vi "DisplacementLogic.vi"   [LabVIEW 2016]
uses:
  DisplacementData.ctl
  DisplacementStates.ctl
  <vilib>/Platform/TimedLoop/XDataNode/timing_clust.ctl
  <vilib>/Platform/TimedLoop/XDataNode/nitl_modes.ctl
  <vilib>/Platform/TimedLoop/XDataNode/wakeup.ctl
  Telemetry/TelemetryFields.ctl
  Telemetry/TelemetryDataTypes.ctl
  Telemetry/TelemetryUpdateModes.ctl
  DisplacementErrorCodes.ctl
  <vilib>/rvi/Emulation/niFpgaSctlEmulationGetInTimedLoop.vi
  <vilib>/rvi/Emulation/niFpgaEmulationReportErrorSimple.vi
  <vilib>/rvi/Emulation/niFpgaGetClockAttributes.vi
  <vilib>/rvi/Emulation/niFpgaCriticalErrorInLSC.vi
  <vilib>/rvi/Emulation/niFpgaEmulationIsFPGAContextNoSignature.vi
  <vilib>/rvi/DataTransferAndStorage/Container/Common/niFpgaContainerGetUniqueNameForEmu.vi
  <vilib>/rvi/Memory/Memory_Emulation/niFpgaMemoryEmulationCacheClearOnFirstRun.vi
  <vilib>/rvi/Memory/Memory_Emulation/nirvimemoryEmulationManagerCache_MakeExclusive.vi
  <vilib>/rvi/Memory/Memory_Emulation/niFpgaMemoryEmulationValidateCache.vi
  <vilib>/rvi/Memory/Memory_Emulation/nirvimemoryEmulationManagerCache_InsertValue.vi
  <vilib>/Utility/error.llb/Clear Errors.vi
  <vilib>/rvi/Memory/Memory_Emulation/nirvimemoryEmulationManagerCache_ReleaseExclusive.vi
  <vilib>/rvi/Memory/Memory_Emulation/nirvimemoryEmulationManagerCache_GetValue.vi
  <vilib>/rvi/Memory/Memory_Emulation/nirvimemoryEmulationManagerCache_SetValue.vi
  <vilib>/rvi/Emulation/niFpgaProcessEmulError.vi
  <vilib>/rvi/errors/niFpgaSetErrorForExecOnDevCompSimple.vi
  <vilib>/rvi/eio/common/nirviEmuReportErrorAndStop.vi
  <vilib>/rvi/FIFO/Fifo_Resource/nirvififoEmulationSetSize.vi
  <vilib>/rvi/FIFO/Fifo_Resource/nirviFifoEmulationQueueMgr.vi
  <instcachedir>/0/nirviFifoEmulationQueueMgr_E5CAEC123FF24DC58D834DCA3CDAA9B5.lvgen/nirviFifoEmulationQueueMgr_E5CAEC123FF24DC58D834DCA3CDAA9B5_009.vi
  <vilib>/rvi/FIFO/Fifo_Resource/nirvififoEmulationDetermineInputValidOut.vi
  <vilib>/rvi/FIFO/Fifo_Resource/nirvififoEmulationCreateLock.vi
  <vilib>/rvi/FIFO/Fifo_Resource/nirvififoEmulationObtainLock.vi
  <vilib>/rvi/FIFO/Fifo_Resource/nirvififoEmulationReleaseLock.vi
  <vilib>/rvi/occurrence/nirviWaitOnOccurrenceBase.vi
  <vilib>/rvi/errors/nirviReportUnexpectedCaseInternalError.vi
  <vilib>/rvi/errors/nirviReportUnexpectedCaseInternalError (U32).vi
  <instcachedir>/0/nirviFifoEmulationQueueMgr_E5CAEC123FF24DC58D834DCA3CDAA9B5.lvgen/nirviFifoEmulationQueueMgr_E5CAEC123FF24DC58D834DCA3CDAA9B5_024.vi
  <vilib>/rvi/eio/common/nirviEmuTemplateMethod_errors.vi
  <vilib>/Platform/TimedLoop/XDataNode/XDataNode.xnode
  <vilib>/rvi/DataTransferAndStorage/Container/XNode/niFpgaContainer.xnode
  <vilib>/rvi/DataTransferAndStorage/Register/Emulation/niFpgaRegisterEmulation.vi
  <vilib>/rvi/FIFO/Fifo_Resource/nirvififoEmulationWrite.vi
  <vilib>/rvi/FIFO/Fifo_Resource/nirvififoEmulationRead.vi
  <vilib>/eio/EIONode/EIONode.xnode
  <vilib>/Platform/TimedLoop/XDataNode/XDNodeRunTimeDep.lvlib
types:
  T1 = typedef "DisplacementData.ctl" = cluster{"State":T2, "Flags":u8, "Sensor":u8, "Timestamp":u64, "Negative":bool, "Sensor1":i32, "Sensor2":i32, "Sensor3":i32, "Sensor4":i32, "Sensor5":i32, "Sensor6":i32, "Sensor7":i32, "Sensor8":i32}
  T2 = typedef "DisplacementStates.ctl" = enum16{"WaitForTrigger", "ClearRxFIFO", "WaitForClearComplete", "WriteM", "Write0", "WriteCR", "WriteNL", "ReadFirstCharacter", "ReadDataResponse", "ReadDeliminator", "ReadSign", "ReadHundreds", "ReadTens", "ReadOnes", "ReadDecimal", "ReadTenths", "ReadHundredths", "ReadThousandths", "ReadTenThousandths", "StartMoveData", "MoveTimestamp", "MoveData", "ReadErrorResponse", "ResponseUnknownError", "ResponseInvalidError"}
  T3 = typedef "XDNodeRunTimeDep.lvlib/timing_clust.ctl" = cluster{"Expected End [f-1]":u64, "Actual End [f-1]":u64, "Finished Late? [f-1]":bool, "Expected End [i-1]":u64, "Actual End [i-1]":u64, "Finished Late? [i-1]":bool, "Expected Start [i]":u64, "Actual Start [i]":u64, "Expected Start [f]":u64, "Actual Start [f]":u64, "Source Name":string, "Structure Name":string, "Period":i64, "Deadline":i64, "Offset":i64, "Start":i64, "Priority":i32, "Timeout":i32, "Mode":T4, "Wakeup Reason":T5, "Error":errorcluster, "Source Type":string, "Secondary Source Type":string, "Global End Time":u64, "Global Start Time":u64, "Frame Duration":u64, "Iteration Duration":u64, "Assigned CPU":i32, "I/O Scan Engine Mode":u32}
  T4 = typedef "XDNodeRunTimeDep.lvlib/nitl_modes.ctl" = enum32{"No Change", "Process missed periods, maintain original phase", "Discard missed periods, maintain original phase", "Process missed periods, ignore original phase", "Discard missed periods, ignore original phase"}
  T5 = typedef "XDNodeRunTimeDep.lvlib/wakeup.ctl" = enum32{"Normal", "Aborted", "Asynchronous wakeup", "Timing source error", "Timed loop error", "Timeout"}
  T6 = typedef "TelemetryUpdateModes.ctl" = enum8{"=", "+", "-", "|"}
  T7 = typedef "TelemetryDataTypes.ctl" = enum8{"U8", "U16", "U32", "U64", "I8", "I16", "I32", "I64", "SGL"}
  T8 = typedef "TelemetryFields.ctl" = enum16{"InclinometerErrorCode", "InclinometerTxBytes", "InclinometerRxBytes", "InclinometerTxFrames", "InclinometerRxFrames", "InclinometerTimestamp", "InclinometerAngle", "DisplacementErrorCode", "DisplacementTxBytes", "DisplacementRxBytes", "DisplacementTxFrames", "DisplacementRxFrames", "DisplacementTimestamp", "Displacement1", "Displacement2", "Displacement3", "Displacement4", "Displacement5", "Displacement6", "Displacement7", "Displacement8", "AccelerometerSampleCount", "AccelerometerTimestamp", "AccelerometerRaw1", "AccelerometerRaw2", "AccelerometerRaw3", "AccelerometerRaw4", "AccelerometerRaw5", "AccelerometerRaw6", "AccelerometerRaw7", "AccelerometerRaw8", "AccelerometerEng1", "AccelerometerEng2", "AccelerometerEng3", "AccelerometerEng4", "AccelerometerEng5", "AccelerometerEng6", "AccelerometerEng7", "AccelerometerEng8", "AngularAccelerationX", "AngularAccelerationY", "AngularAccelerationZ"}
  T9 = typedef "TelemetryUpdateData.ctl" = cluster{"DataType":T7, "Mode":T6, "Field":T8, "Data":u64}
  T10 = typedef "DisplacementErrorCodes.ctl" = u8
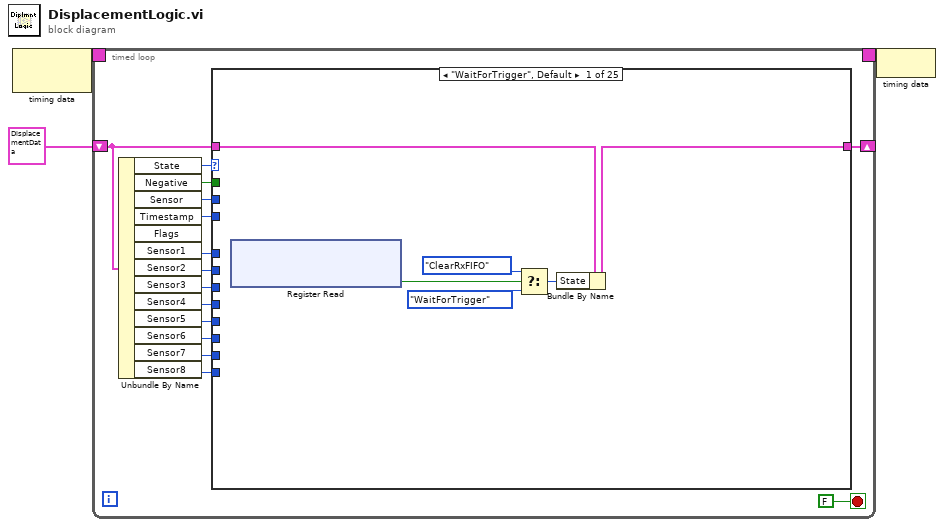
[diagram p0: block diagram]
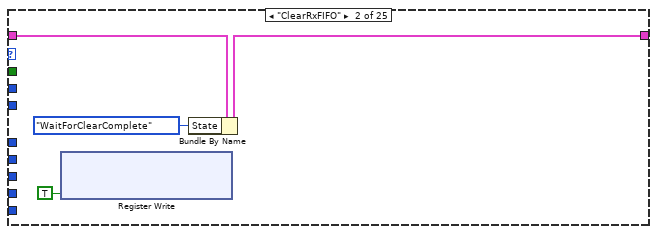
[diagram p2: hidden frame]
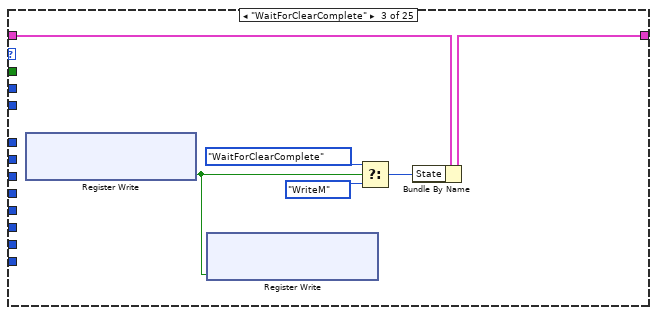
[diagram p3: hidden frame]
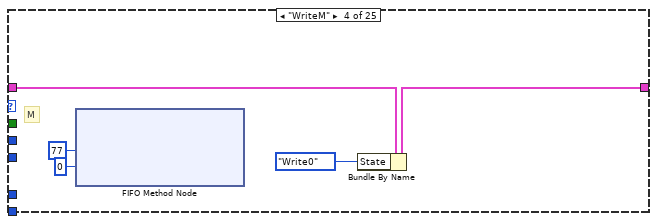
[diagram p4: hidden frame]
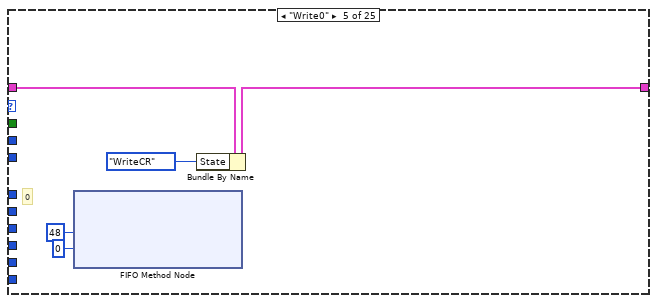
[diagram p5: hidden frame]
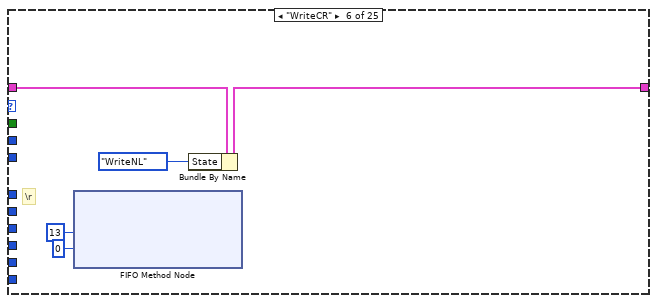
[diagram p6: hidden frame]
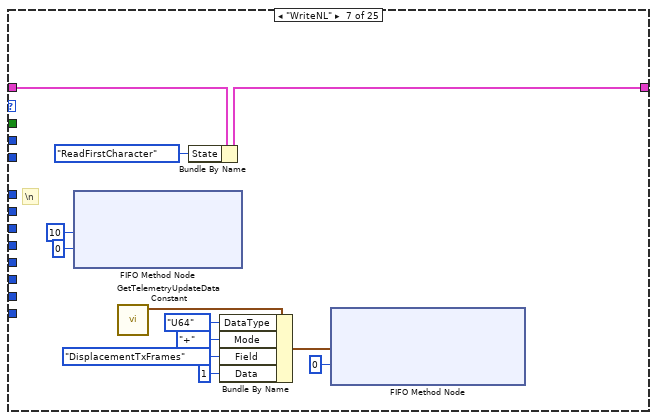
[diagram p7: hidden frame]
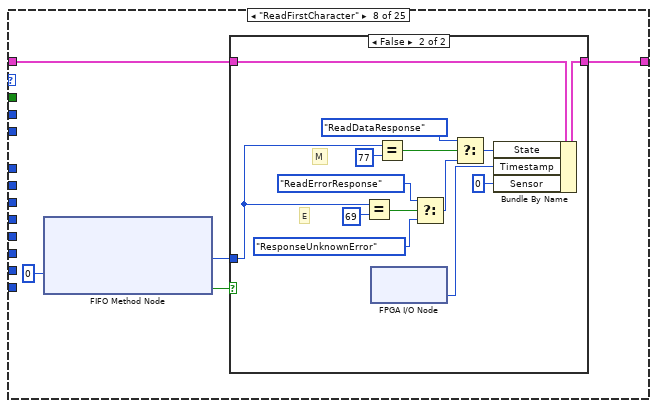
[diagram p8: hidden frame]
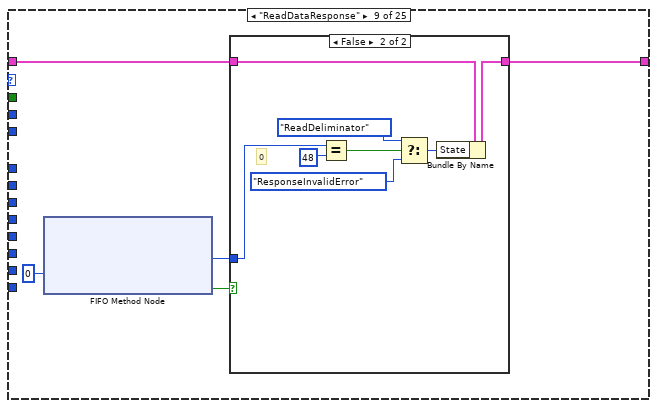
[diagram p10: hidden frame]
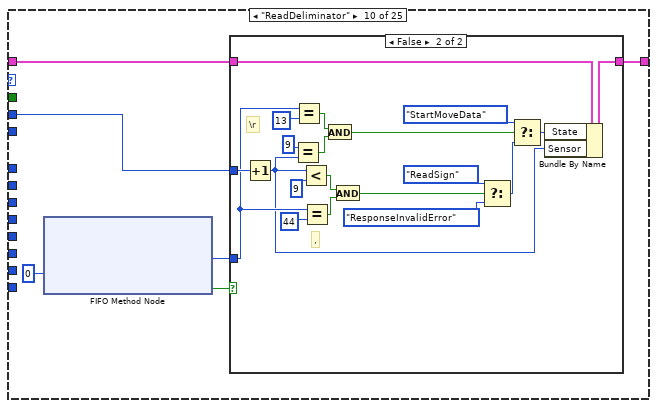
[diagram p12: hidden frame]
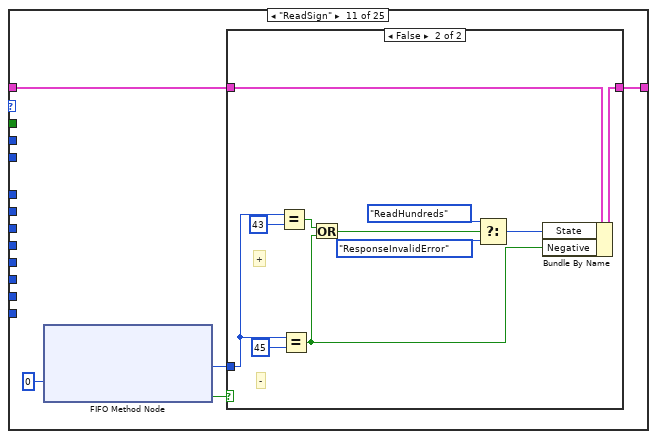
[diagram p14: hidden frame]
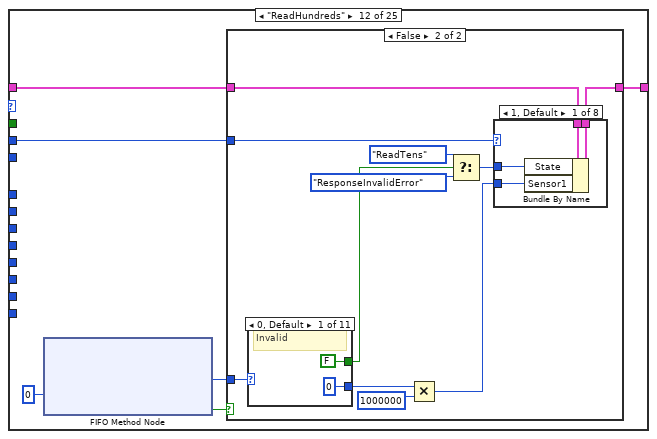
[diagram p16: hidden frame]
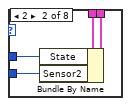
[diagram p18: hidden frame]
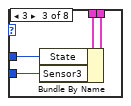
[diagram p19: hidden frame]
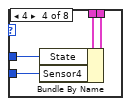
[diagram p20: hidden frame]
diagram:
  n1 = node-c288() -> (w3:T3)  [unwired: 1 in]
  n2 = timed-loop {
    timing: w3 -> [_]
    timing-out: [_] -> w2
    shift-right: [w18] -> _
    shift-left: T1 {"State"=enum."WaitForTrigger", "Flags"=0, "Sensor"=0, "Timestamp"=0, "Negative"=FALSE, "Sensor1"=0, "Sensor2"=0, "Sensor3"=0, "Sensor4"=0, "Sensor5"=0, "Sensor6"=0, "Sensor7"=0, "Sensor8"=0} ("DisplacementData") -> [w17]
    stop <- FALSE stop-if-true
    n3 = Unbundle By Name(w17) -> ("State"=w16:T2, "Negative"=w4:bool, "Sensor"=w7:u8, "Timestamp"=w5:u64, "Sensor1"=w15:i32, "Sensor2"=w14:i32, "Sensor3"=w13:i32, "Sensor4"=w12:i32, "Sensor5"=w11:i32, "Sensor6"=w10:i32, "Sensor7"=w9:i32, "Sensor8"=w8:i32)  [unwired: 1 out]
    n4 = case shown="\"WaitForTrigger\", Default" w16 {
      tunnel: [w20 w26 w33 w38 w43 w48 w60 w65 w85 w100 w126 w144 w225 w316 w397 w421 w512 w603 w695 w787 w798 w822 w841 w851 w861] -> w18
      tunnel: w17 -> [w23 w27 w34 w39 w44 w49 w61 w66 w86 w101 w127 w145 w226 w317 w398 w422 w513 w604 w696 w788 w799 w823 w842 w852 w862]
      tunnel: w15 -> [_ _ _ _ _ _ _ _ _ _ _ _ w220 w311 _ w416 w507 w598 w690 _ _ w821 _ _ _]
      tunnel: w14 -> [_ _ _ _ _ _ _ _ _ _ _ _ w219 w310 _ w415 w506 w597 w689 _ _ w820 _ _ _]
      tunnel: w13 -> [_ _ _ _ _ _ _ _ _ _ _ _ w218 w309 _ w414 w505 w596 w688 _ _ w819 _ _ _]
      tunnel: w12 -> [_ _ _ _ _ _ _ _ _ _ _ _ w217 w308 _ w413 w504 w595 w687 _ _ w818 _ _ _]
      tunnel: w11 -> [_ _ _ _ _ _ _ _ _ _ _ _ w216 w307 _ w412 w503 w594 w686 _ _ w817 _ _ _]
      tunnel: w10 -> [_ _ _ _ _ _ _ _ _ _ _ _ w215 w306 _ w411 w502 w593 w685 _ _ w816 _ _ _]
      tunnel: w9 -> [_ _ _ _ _ _ _ _ _ _ _ _ w214 w305 _ w410 w501 w592 w684 _ _ w815 _ _ _]
      tunnel: w8 -> [_ _ _ _ _ _ _ _ _ _ _ _ w213 w304 _ w409 w500 w591 w683 _ _ w814 _ _ _]
      tunnel: w7 -> [_ _ _ _ _ _ _ _ _ w96 _ w140 w221 w312 _ w417 w508 w599 w691 _ _ w807 _ _ _]
      tunnel: w5 -> [_ _ _ _ _ _ _ _ _ _ _ _ _ _ _ _ _ _ _ _ w789 _ _ _ _]
      tunnel: w4 -> [_ _ _ _ _ _ _ _ _ _ _ _ _ _ _ _ _ _ w681 _ _ _ _ _ _]
      frame "WaitForTrigger", Default {
        n5 = xnode ("Register Read")() -> ("Data"=w24:bool)  [unwired: 1 in, 1 out]
        n6 = Select(t=DisplacementStates."ClearRxFIFO" ("DisplacementStates"), s=w24, f=DisplacementStates."WaitForTrigger") -> (s? t:f=w21:T2)
        n7 = Bundle By Name(cluster=w23, "State"=w21) -> (w20:T1)
      }
      frame "ClearRxFIFO" {
        n8 = xnode ("Register Write")("Data"=TRUE) -> ()  [unwired: 1 in, 1 out]
        n9 = Bundle By Name(cluster=w27, "State"=DisplacementStates."WaitForClearComplete") -> (w26:T1)
      }
      frame "WaitForClearComplete" {
        n10 = xnode ("Register Write")() -> ("Data"=w30:bool)  [unwired: 1 in, 1 out]
        n11 = xnode ("Register Write")("Data"=w30) -> ()  [unwired: 1 in, 1 out]
        n12 = Select(t=DisplacementStates."WaitForClearComplete" ("State"), s=w30, f=DisplacementStates."WriteM") -> (s? t:f=w31:T2)
        n13 = Bundle By Name(cluster=w34, "State"=w31) -> (w33:T1)
      }
      frame "WriteM" {
        # "M"
        n14 = xnode ("FIFO Method Node")("Element"=u8 77, "Timeout"=0) -> ()  [unwired: 1 in, 2 out]
        n15 = Bundle By Name(cluster=w39, "State"=DisplacementStates."Write0" ("f")) -> (w38:T1)
      }
      frame "Write0" {
        # "0"
        n16 = xnode ("FIFO Method Node")("Element"=u8 48, "Timeout"=0) -> ()  [unwired: 1 in, 2 out]
        n17 = Bundle By Name(cluster=w44, "State"=DisplacementStates."WriteCR" ("f")) -> (w43:T1)
      }
      frame "WriteCR" {
        # "\\r"
        n18 = xnode ("FIFO Method Node")("Element"=u8 13, "Timeout"=0) -> ()  [unwired: 1 in, 2 out]
        n19 = Bundle By Name(cluster=w49, "State"=DisplacementStates."WriteNL" ("f")) -> (w48:T1)
      }
      frame "WriteNL" {
        # "\\n"
        n20 = xnode ("FIFO Method Node")("Element"=u8 10, "Timeout"=0) -> ()  [unwired: 1 in, 2 out]
        n21 = call "GetTelemetryUpdateDataConstant.vi"() -> ("TelemetryUpdateData"=w55:T9)  [unwired: 11 in]
        n22 = Bundle By Name(cluster=w61, "State"=DisplacementStates."ReadFirstCharacter") -> (w60:T1)
        n23 = Bundle By Name(cluster=w55, "DataType"=TelemetryDataTypes."U64" ("TelemetryDataTypes"), "Mode"=TelemetryUpdateModes."+" ("TelemetryUpdateModes"), "Field"=TelemetryFields."DisplacementTxFrames", "Data"=u64 1) -> (w50:T9)
        n24 = xnode ("FIFO Method Node")("Element"=w50, "Timeout"=0) -> ()  [unwired: 1 in, 2 out]
      }
      frame "ReadFirstCharacter" {
        n25 = xnode ("FIFO Method Node")("Timeout"=0) -> ("Element"=w62:u8, "Timed Out?"=w63:bool)  [unwired: 1 in, 1 out]
        n26 = case shown="False" w63 {
          tunnel: w66 -> [w67 w81]
          tunnel: [w67 w80] -> w65
          tunnel: w62 -> [_ w73]
          frame True {
          }
          frame False {
            # "E"
            # "M"
            n27 = Equal?(x=w73, y=u8 69) -> (x = y?=w74:bool)
            n28 = xnode "FPGA I/O Node"() -> ("Time"=w69:u64)  [unwired: 1 in, 1 out]
            n29 = Equal?(x=w73, y=u8 77) -> (x = y?=w78:bool)
            n30 = Select(t=DisplacementStates."ReadErrorResponse" ("State"), s=w74, f=DisplacementStates."ResponseUnknownError") -> (s? t:f=w71:T2)
            n31 = Select(t=DisplacementStates."ReadDataResponse" ("State"), s=w78, f=w71) -> (s? t:f=w77:T2)
            n32 = Bundle By Name(cluster=w81, "State"=w77, "Timestamp"=w69, "Sensor"=u8 0) -> (w80:T1)
          }
        }
      }
      frame "ReadDataResponse" {
        n33 = xnode ("FIFO Method Node")("Timeout"=0) -> ("Element"=w82:u8, "Timed Out?"=w83:bool)  [unwired: 1 in, 1 out]
        n34 = case shown="False" w83 {
          tunnel: w86 -> [w87 w95]
          tunnel: [w87 w94] -> w85
          tunnel: w82 -> [_ w89]
          frame True {
          }
          frame False {
            # "0"
            n35 = Equal?(x=w89, y=u8 48) -> (x = y?=w92:bool)
            n36 = Select(t=DisplacementStates."ReadDeliminator" ("State"), s=w92, f=DisplacementStates."ResponseInvalidError") -> (s? t:f=w91:T2)
            n37 = Bundle By Name(cluster=w95, "State"=w91) -> (w94:T1)
          }
        }
      }
      frame "ReadDeliminator" {
        n38 = xnode ("FIFO Method Node")("Timeout"=0) -> ("Element"=w97:u8, "Timed Out?"=w98:bool)  [unwired: 1 in, 1 out]
        n39 = case shown="False" w98 {
          tunnel: w101 -> [w102 w122]
          tunnel: [w102 w121] -> w100
          tunnel: w97 -> [_ w111]
          tunnel: w96 -> [_ w118]
          frame True {
          }
          frame False {
            # "\\r"
            # ","
            n40 = Increment(x=w118) -> (x+1=w103:u8)
            n41 = Equal?(x=u8 9, y=w103) -> (x = y?=w110:bool)
            n42 = Equal?(x=w111, y=u8 13) -> (x = y?=w109:bool)
            n43 = Less?(x=w103, y=u8 9) -> (x < y?=w116:bool)
            n44 = Equal?(x=w111, y=u8 44) -> (x = y?=w115:bool)
            n45 = And(x=w109, y=w110) -> (x .and. y?=w107:bool)
            n46 = And(x=w116, y=w115) -> (x .and. y?=w104:bool)
            n47 = Select(t=DisplacementStates."ReadSign" ("State"), s=w104, f=DisplacementStates."ResponseInvalidError") -> (s? t:f=w108:T2)
            n48 = Select(t=DisplacementStates."StartMoveData", s=w107, f=w108) -> (s? t:f=w105:T2)
            n49 = Bundle By Name(cluster=w122, "State"=w105, "Sensor"=w103) -> (w121:T1)
          }
        }
      }
      frame "ReadSign" {
        n50 = xnode ("FIFO Method Node")("Timeout"=0) -> ("Element"=w123:u8, "Timed Out?"=w124:bool)  [unwired: 1 in, 1 out]
        n51 = case shown="False" w124 {
          tunnel: w127 -> [w128 w139]
          tunnel: [w128 w138] -> w126
          tunnel: w123 -> [_ w135]
          frame True {
          }
          frame False {
            # "+"
            # "-"
            n52 = Equal?(x=w135, y=u8 43) -> (x = y?=w136:bool)
            n53 = Equal?(x=w135, y=u8 45) -> (x = y?=w133:bool)
            n54 = Or(x=w136, y=w133) -> (x .or. y?=w132:bool)
            n55 = Select(t=DisplacementStates."ReadHundreds" ("State"), s=w132, f=DisplacementStates."ResponseInvalidError") -> (s? t:f=w130:T2)
            n56 = Bundle By Name(cluster=w139, "State"=w130, "Negative"=w133) -> (w138:T1)
          }
        }
      }
      frame "ReadHundreds" {
        n57 = xnode ("FIFO Method Node")("Timeout"=0) -> ("Element"=w141:u8, "Timed Out?"=w142:bool)  [unwired: 1 in, 1 out]
        n58 = case shown="False" w142 {
          tunnel: w145 -> [w146 w157]
          tunnel: [w146 w156] -> w144
          tunnel: w141 -> [_ w155]
          tunnel: w140 -> [_ w152]
          frame True {
          }
          frame False {
            n59 = case shown="0, Default" w155 {
              tunnel: [0 0 1 2 3 4 5 6 7 8 9] -> w154
              tunnel: [FALSE TRUE TRUE TRUE TRUE TRUE TRUE TRUE TRUE TRUE TRUE] -> w151
              frame 0, Default {
                # "Invalid"
              }
              frame 48 {
                # "0"
              }
              frame 49 {
                # "1"
              }
              frame 50 {
                # "2"
              }
              frame 51 {
                # "3"
              }
              frame 52 {
                # "4"
              }
              frame 53 {
                # "5"
              }
              frame 54 {
                # "6"
              }
              frame 55 {
                # "7"
              }
              frame 56 {
                # "8"
              }
              frame 57 {
                # "9"
              }
            }
            n60 = Multiply(x=w154, y=1000000) -> (x*y=w147:i32)
            n61 = Select(t=DisplacementStates."ReadTens" ("State"), s=w151, f=DisplacementStates."ResponseInvalidError" ("State")) -> (s? t:f=w150:T2)
            n62 = case shown="1, Default" w152 {
              tunnel: w157 -> [w161 w165 w169 w173 w177 w181 w185 w189]
              tunnel: [w160 w164 w168 w172 w176 w180 w184 w188] -> w156
              tunnel: w150 -> [w159 w163 w167 w171 w175 w179 w183 w187]
              tunnel: w147 -> [w158 w162 w166 w170 w174 w178 w182 w186]
              frame 1, Default {
                n63 = Bundle By Name(cluster=w161, "State"=w159, "Sensor1"=w158) -> (w160:T1)
              }
              frame 2 {
                n64 = Bundle By Name(cluster=w165, "State"=w163, "Sensor2"=w162) -> (w164:T1)
              }
              frame 3 {
                n65 = Bundle By Name(cluster=w169, "State"=w167, "Sensor3"=w166) -> (w168:T1)
              }
              frame 4 {
                n66 = Bundle By Name(cluster=w173, "State"=w171, "Sensor4"=w170) -> (w172:T1)
              }
              frame 5 {
                n67 = Bundle By Name(cluster=w177, "State"=w175, "Sensor5"=w174) -> (w176:T1)
              }
              frame 6 {
                n68 = Bundle By Name(cluster=w181, "State"=w179, "Sensor6"=w178) -> (w180:T1)
              }
              frame 7 {
                n69 = Bundle By Name(cluster=w185, "State"=w183, "Sensor7"=w182) -> (w184:T1)
              }
              frame 8 {
                n70 = Bundle By Name(cluster=w189, "State"=w187, "Sensor8"=w186) -> (w188:T1)
              }
            }
          }
        }
      }
      frame "ReadTens" {
        n71 = case shown="1, Default" w221 {
          tunnel: w220 -> [w227 _ _ _ _ _ _ _]
          tunnel: w219 -> [_ w228 _ _ _ _ _ _]
          tunnel: w218 -> [_ _ w229 _ _ _ _ _]
          tunnel: w217 -> [_ _ _ w230 _ _ _ _]
          tunnel: w216 -> [_ _ _ _ w231 _ _ _]
          tunnel: w215 -> [_ _ _ _ _ w232 _ _]
          tunnel: w214 -> [_ _ _ _ _ _ w233 _]
          tunnel: w213 -> [_ _ _ _ _ _ _ w234]
          tunnel: [w227 w228 w229 w230 w231 w232 w233 w234] -> w212
          frame 1, Default {
          }
          frame 2 {
          }
          frame 3 {
          }
          frame 4 {
          }
          frame 5 {
          }
          frame 6 {
          }
          frame 7 {
          }
          frame 8 {
          }
        }
        n72 = xnode ("FIFO Method Node")("Timeout"=0) -> ("Element"=w222:u8, "Timed Out?"=w223:bool)  [unwired: 1 in, 1 out]
        n73 = case shown="False" w223 {
          tunnel: w226 -> [w235 w248]
          tunnel: [w235 w247] -> w225
          tunnel: w222 -> [_ w246]
          tunnel: w221 -> [_ w243]
          tunnel: w212 -> [_ w238]
          frame True {
          }
          frame False {
            n74 = case shown="0, Default" w246 {
              tunnel: [0 0 1 2 3 4 5 6 7 8 9] -> w245
              tunnel: [FALSE TRUE TRUE TRUE TRUE TRUE TRUE TRUE TRUE TRUE TRUE] -> w242
              frame 0, Default {
                # "Invalid"
              }
              frame 48 {
                # "0"
              }
              frame 49 {
                # "1"
              }
              frame 50 {
                # "2"
              }
              frame 51 {
                # "3"
              }
              frame 52 {
                # "4"
              }
              frame 53 {
                # "5"
              }
              frame 54 {
                # "6"
              }
              frame 55 {
                # "7"
              }
              frame 56 {
                # "8"
              }
              frame 57 {
                # "9"
              }
            }
            n75 = Multiply(x=w245, y=100000) -> (x*y=w237:i32)
            n76 = Add(x=w238, y=w237) -> (x+y=w236:i32)
            n77 = Select(t=DisplacementStates."ReadOnes" ("State"), s=w242, f=DisplacementStates."ResponseInvalidError" ("State")) -> (s? t:f=w241:T2)
            n78 = case shown="1, Default" w243 {
              tunnel: w248 -> [w252 w256 w260 w264 w268 w272 w276 w280]
              tunnel: [w251 w255 w259 w263 w267 w271 w275 w279] -> w247
              tunnel: w241 -> [w250 w254 w258 w262 w266 w270 w274 w278]
              tunnel: w236 -> [w249 w253 w257 w261 w265 w269 w273 w277]
              frame 1, Default {
                n79 = Bundle By Name(cluster=w252, "State"=w250, "Sensor1"=w249) -> (w251:T1)
              }
              frame 2 {
                n80 = Bundle By Name(cluster=w256, "State"=w254, "Sensor2"=w253) -> (w255:T1)
              }
              frame 3 {
                n81 = Bundle By Name(cluster=w260, "State"=w258, "Sensor3"=w257) -> (w259:T1)
              }
              frame 4 {
                n82 = Bundle By Name(cluster=w264, "State"=w262, "Sensor4"=w261) -> (w263:T1)
              }
              frame 5 {
                n83 = Bundle By Name(cluster=w268, "State"=w266, "Sensor5"=w265) -> (w267:T1)
              }
              frame 6 {
                n84 = Bundle By Name(cluster=w272, "State"=w270, "Sensor6"=w269) -> (w271:T1)
              }
              frame 7 {
                n85 = Bundle By Name(cluster=w276, "State"=w274, "Sensor7"=w273) -> (w275:T1)
              }
              frame 8 {
                n86 = Bundle By Name(cluster=w280, "State"=w278, "Sensor8"=w277) -> (w279:T1)
              }
            }
          }
        }
      }
      frame "ReadOnes" {
        n87 = case shown="1, Default" w312 {
          tunnel: w311 -> [w318 _ _ _ _ _ _ _]
          tunnel: w310 -> [_ w319 _ _ _ _ _ _]
          tunnel: w309 -> [_ _ w320 _ _ _ _ _]
          tunnel: w308 -> [_ _ _ w321 _ _ _ _]
          tunnel: w307 -> [_ _ _ _ w322 _ _ _]
          tunnel: w306 -> [_ _ _ _ _ w323 _ _]
          tunnel: w305 -> [_ _ _ _ _ _ w324 _]
          tunnel: w304 -> [_ _ _ _ _ _ _ w325]
          tunnel: [w318 w319 w320 w321 w322 w323 w324 w325] -> w303
          frame 1, Default {
          }
          frame 2 {
          }
          frame 3 {
          }
          frame 4 {
          }
          frame 5 {
          }
          frame 6 {
          }
          frame 7 {
          }
          frame 8 {
          }
        }
        n88 = xnode ("FIFO Method Node")("Timeout"=0) -> ("Element"=w313:u8, "Timed Out?"=w314:bool)  [unwired: 1 in, 1 out]
        n89 = case shown="False" w314 {
          tunnel: w317 -> [w326 w339]
          tunnel: [w326 w338] -> w316
          tunnel: w313 -> [_ w337]
          tunnel: w312 -> [_ w334]
          tunnel: w303 -> [_ w329]
          frame True {
          }
          frame False {
            n90 = case shown="0, Default" w337 {
              tunnel: [0 0 1 2 3 4 5 6 7 8 9] -> w336
              tunnel: [FALSE TRUE TRUE TRUE TRUE TRUE TRUE TRUE TRUE TRUE TRUE] -> w333
              frame 0, Default {
                # "Invalid"
              }
              frame 48 {
                # "0"
              }
              frame 49 {
                # "1"
              }
              frame 50 {
                # "2"
              }
              frame 51 {
                # "3"
              }
              frame 52 {
                # "4"
              }
              frame 53 {
                # "5"
              }
              frame 54 {
                # "6"
              }
              frame 55 {
                # "7"
              }
              frame 56 {
                # "8"
              }
              frame 57 {
                # "9"
              }
            }
            n91 = Multiply(x=w336, y=10000) -> (x*y=w328:i32)
            n92 = Add(x=w329, y=w328) -> (x+y=w327:i32)
            n93 = Select(t=DisplacementStates."ReadDecimal" ("State"), s=w333, f=DisplacementStates."ResponseInvalidError" ("State")) -> (s? t:f=w332:T2)
            n94 = case shown="1, Default" w334 {
              tunnel: w339 -> [w343 w347 w351 w355 w359 w363 w367 w371]
              tunnel: [w342 w346 w350 w354 w358 w362 w366 w370] -> w338
              tunnel: w332 -> [w341 w345 w349 w353 w357 w361 w365 w369]
              tunnel: w327 -> [w340 w344 w348 w352 w356 w360 w364 w368]
              frame 1, Default {
                n95 = Bundle By Name(cluster=w343, "State"=w341, "Sensor1"=w340) -> (w342:T1)
              }
              frame 2 {
                n96 = Bundle By Name(cluster=w347, "State"=w345, "Sensor2"=w344) -> (w346:T1)
              }
              frame 3 {
                n97 = Bundle By Name(cluster=w351, "State"=w349, "Sensor3"=w348) -> (w350:T1)
              }
              frame 4 {
                n98 = Bundle By Name(cluster=w355, "State"=w353, "Sensor4"=w352) -> (w354:T1)
              }
              frame 5 {
                n99 = Bundle By Name(cluster=w359, "State"=w357, "Sensor5"=w356) -> (w358:T1)
              }
              frame 6 {
                n100 = Bundle By Name(cluster=w363, "State"=w361, "Sensor6"=w360) -> (w362:T1)
              }
              frame 7 {
                n101 = Bundle By Name(cluster=w367, "State"=w365, "Sensor7"=w364) -> (w366:T1)
              }
              frame 8 {
                n102 = Bundle By Name(cluster=w371, "State"=w369, "Sensor8"=w368) -> (w370:T1)
              }
            }
          }
        }
      }
      frame "ReadDecimal" {
        n103 = xnode ("FIFO Method Node")("Timeout"=0) -> ("Element"=w394:u8, "Timed Out?"=w395:bool)  [unwired: 1 in, 1 out]
        n104 = case shown="False" w395 {
          tunnel: w398 -> [w399 w407]
          tunnel: [w399 w406] -> w397
          tunnel: w394 -> [_ w402]
          frame True {
          }
          frame False {
            # "."
            n105 = Equal?(x=w402, y=u8 46) -> (x = y?=w400:bool)
            n106 = Select(t=DisplacementStates."ReadTenths" ("State"), s=w400, f=DisplacementStates."ResponseInvalidError" ("State")) -> (s? t:f=w405:T2)
            n107 = Bundle By Name(cluster=w407, "State"=w405) -> (w406:T1)
          }
        }
      }
      frame "ReadTenths" {
        n108 = case shown="1, Default" w417 {
          tunnel: w416 -> [w423 _ _ _ _ _ _ _]
          tunnel: w415 -> [_ w424 _ _ _ _ _ _]
          tunnel: w414 -> [_ _ w425 _ _ _ _ _]
          tunnel: w413 -> [_ _ _ w426 _ _ _ _]
          tunnel: w412 -> [_ _ _ _ w427 _ _ _]
          tunnel: w411 -> [_ _ _ _ _ w428 _ _]
          tunnel: w410 -> [_ _ _ _ _ _ w429 _]
          tunnel: w409 -> [_ _ _ _ _ _ _ w430]
          tunnel: [w423 w424 w425 w426 w427 w428 w429 w430] -> w408
          frame 1, Default {
          }
          frame 2 {
          }
          frame 3 {
          }
          frame 4 {
          }
          frame 5 {
          }
          frame 6 {
          }
          frame 7 {
          }
          frame 8 {
          }
        }
        n109 = xnode ("FIFO Method Node")("Timeout"=0) -> ("Element"=w418:u8, "Timed Out?"=w419:bool)  [unwired: 1 in, 1 out]
        n110 = case shown="False" w419 {
          tunnel: w422 -> [w431 w444]
          tunnel: [w431 w443] -> w421
          tunnel: w418 -> [_ w442]
          tunnel: w417 -> [_ w439]
          tunnel: w408 -> [_ w434]
          frame True {
          }
          frame False {
            n111 = case shown="0, Default" w442 {
              tunnel: [0 0 1 2 3 4 5 6 7 8 9] -> w441
              tunnel: [FALSE TRUE TRUE TRUE TRUE TRUE TRUE TRUE TRUE TRUE TRUE] -> w438
              frame 0, Default {
                # "Invalid"
              }
              frame 48 {
                # "0"
              }
              frame 49 {
                # "1"
              }
              frame 50 {
                # "2"
              }
              frame 51 {
                # "3"
              }
              frame 52 {
                # "4"
              }
              frame 53 {
                # "5"
              }
              frame 54 {
                # "6"
              }
              frame 55 {
                # "7"
              }
              frame 56 {
                # "8"
              }
              frame 57 {
                # "9"
              }
            }
            n112 = Multiply(x=w441, y=1000) -> (x*y=w433:i32)
            n113 = Add(x=w434, y=w433) -> (x+y=w432:i32)
            n114 = Select(t=DisplacementStates."ReadHundredths" ("State"), s=w438, f=DisplacementStates."ResponseInvalidError" ("State")) -> (s? t:f=w437:T2)
            n115 = case shown="1, Default" w439 {
              tunnel: w444 -> [w448 w452 w456 w460 w464 w468 w472 w476]
              tunnel: [w447 w451 w455 w459 w463 w467 w471 w475] -> w443
              tunnel: w437 -> [w446 w450 w454 w458 w462 w466 w470 w474]
              tunnel: w432 -> [w445 w449 w453 w457 w461 w465 w469 w473]
              frame 1, Default {
                n116 = Bundle By Name(cluster=w448, "State"=w446, "Sensor1"=w445) -> (w447:T1)
              }
              frame 2 {
                n117 = Bundle By Name(cluster=w452, "State"=w450, "Sensor2"=w449) -> (w451:T1)
              }
              frame 3 {
                n118 = Bundle By Name(cluster=w456, "State"=w454, "Sensor3"=w453) -> (w455:T1)
              }
              frame 4 {
                n119 = Bundle By Name(cluster=w460, "State"=w458, "Sensor4"=w457) -> (w459:T1)
              }
              frame 5 {
                n120 = Bundle By Name(cluster=w464, "State"=w462, "Sensor5"=w461) -> (w463:T1)
              }
              frame 6 {
                n121 = Bundle By Name(cluster=w468, "State"=w466, "Sensor6"=w465) -> (w467:T1)
              }
              frame 7 {
                n122 = Bundle By Name(cluster=w472, "State"=w470, "Sensor7"=w469) -> (w471:T1)
              }
              frame 8 {
                n123 = Bundle By Name(cluster=w476, "State"=w474, "Sensor8"=w473) -> (w475:T1)
              }
            }
          }
        }
      }
      frame "ReadHundredths" {
        n124 = case shown="1, Default" w508 {
          tunnel: w507 -> [w514 _ _ _ _ _ _ _]
          tunnel: w506 -> [_ w515 _ _ _ _ _ _]
          tunnel: w505 -> [_ _ w516 _ _ _ _ _]
          tunnel: w504 -> [_ _ _ w517 _ _ _ _]
          tunnel: w503 -> [_ _ _ _ w518 _ _ _]
          tunnel: w502 -> [_ _ _ _ _ w519 _ _]
          tunnel: w501 -> [_ _ _ _ _ _ w520 _]
          tunnel: w500 -> [_ _ _ _ _ _ _ w521]
          tunnel: [w514 w515 w516 w517 w518 w519 w520 w521] -> w499
          frame 1, Default {
          }
          frame 2 {
          }
          frame 3 {
          }
          frame 4 {
          }
          frame 5 {
          }
          frame 6 {
          }
          frame 7 {
          }
          frame 8 {
          }
        }
        n125 = xnode ("FIFO Method Node")("Timeout"=0) -> ("Element"=w509:u8, "Timed Out?"=w510:bool)  [unwired: 1 in, 1 out]
        n126 = case shown="False" w510 {
          tunnel: w513 -> [w522 w535]
          tunnel: [w522 w534] -> w512
          tunnel: w509 -> [_ w533]
          tunnel: w508 -> [_ w530]
          tunnel: w499 -> [_ w525]
          frame True {
          }
          frame False {
            n127 = case shown="0, Default" w533 {
              tunnel: [0 0 1 2 3 4 5 6 7 8 9] -> w532
              tunnel: [FALSE TRUE TRUE TRUE TRUE TRUE TRUE TRUE TRUE TRUE TRUE] -> w529
              frame 0, Default {
                # "Invalid"
              }
              frame 48 {
                # "0"
              }
              frame 49 {
                # "1"
              }
              frame 50 {
                # "2"
              }
              frame 51 {
                # "3"
              }
              frame 52 {
                # "4"
              }
              frame 53 {
                # "5"
              }
              frame 54 {
                # "6"
              }
              frame 55 {
                # "7"
              }
              frame 56 {
                # "8"
              }
              frame 57 {
                # "9"
              }
            }
            n128 = Multiply(x=w532, y=100) -> (x*y=w524:i32)
            n129 = Add(x=w525, y=w524) -> (x+y=w523:i32)
            n130 = Select(t=DisplacementStates."ReadThousandths" ("State"), s=w529, f=DisplacementStates."ResponseInvalidError" ("State")) -> (s? t:f=w528:T2)
            n131 = case shown="1, Default" w530 {
              tunnel: w535 -> [w539 w543 w547 w551 w555 w559 w563 w567]
              tunnel: [w538 w542 w546 w550 w554 w558 w562 w566] -> w534
              tunnel: w528 -> [w537 w541 w545 w549 w553 w557 w561 w565]
              tunnel: w523 -> [w536 w540 w544 w548 w552 w556 w560 w564]
              frame 1, Default {
                n132 = Bundle By Name(cluster=w539, "State"=w537, "Sensor1"=w536) -> (w538:T1)
              }
              frame 2 {
                n133 = Bundle By Name(cluster=w543, "State"=w541, "Sensor2"=w540) -> (w542:T1)
              }
              frame 3 {
                n134 = Bundle By Name(cluster=w547, "State"=w545, "Sensor3"=w544) -> (w546:T1)
              }
              frame 4 {
                n135 = Bundle By Name(cluster=w551, "State"=w549, "Sensor4"=w548) -> (w550:T1)
              }
              frame 5 {
                n136 = Bundle By Name(cluster=w555, "State"=w553, "Sensor5"=w552) -> (w554:T1)
              }
              frame 6 {
                n137 = Bundle By Name(cluster=w559, "State"=w557, "Sensor6"=w556) -> (w558:T1)
              }
              frame 7 {
                n138 = Bundle By Name(cluster=w563, "State"=w561, "Sensor7"=w560) -> (w562:T1)
              }
              frame 8 {
                n139 = Bundle By Name(cluster=w567, "State"=w565, "Sensor8"=w564) -> (w566:T1)
              }
            }
          }
        }
      }
      frame "ReadThousandths" {
        n140 = case shown="1, Default" w599 {
          tunnel: w598 -> [w605 _ _ _ _ _ _ _]
          tunnel: w597 -> [_ w606 _ _ _ _ _ _]
          tunnel: w596 -> [_ _ w607 _ _ _ _ _]
          tunnel: w595 -> [_ _ _ w608 _ _ _ _]
          tunnel: w594 -> [_ _ _ _ w609 _ _ _]
          tunnel: w593 -> [_ _ _ _ _ w610 _ _]
          tunnel: w592 -> [_ _ _ _ _ _ w611 _]
          tunnel: w591 -> [_ _ _ _ _ _ _ w612]
          tunnel: [w605 w606 w607 w608 w609 w610 w611 w612] -> w590
          frame 1, Default {
          }
          frame 2 {
          }
          frame 3 {
          }
          frame 4 {
          }
          frame 5 {
          }
          frame 6 {
          }
          frame 7 {
          }
          frame 8 {
          }
        }
        n141 = xnode ("FIFO Method Node")("Timeout"=0) -> ("Element"=w600:u8, "Timed Out?"=w601:bool)  [unwired: 1 in, 1 out]
        n142 = case shown="False" w601 {
          tunnel: w604 -> [w613 w626]
          tunnel: [w613 w625] -> w603
          tunnel: w600 -> [_ w624]
          tunnel: w599 -> [_ w621]
          tunnel: w590 -> [_ w616]
          frame True {
          }
          frame False {
            n143 = case shown="0, Default" w624 {
              tunnel: [0 0 1 2 3 4 5 6 7 8 9] -> w623
              tunnel: [FALSE TRUE TRUE TRUE TRUE TRUE TRUE TRUE TRUE TRUE TRUE] -> w620
              frame 0, Default {
                # "Invalid"
              }
              frame 48 {
                # "0"
              }
              frame 49 {
                # "1"
              }
              frame 50 {
                # "2"
              }
              frame 51 {
                # "3"
              }
              frame 52 {
                # "4"
              }
              frame 53 {
                # "5"
              }
              frame 54 {
                # "6"
              }
              frame 55 {
                # "7"
              }
              frame 56 {
                # "8"
              }
              frame 57 {
                # "9"
              }
            }
            n144 = Multiply(x=w623, y=10) -> (x*y=w615:i32)
            n145 = Add(x=w616, y=w615) -> (x+y=w614:i32)
            n146 = Select(t=DisplacementStates."ReadTenThousandths" ("State"), s=w620, f=DisplacementStates."ResponseInvalidError" ("State")) -> (s? t:f=w619:T2)
            n147 = case shown="1, Default" w621 {
              tunnel: w626 -> [w630 w634 w638 w642 w646 w650 w654 w658]
              tunnel: [w629 w633 w637 w641 w645 w649 w653 w657] -> w625
              tunnel: w619 -> [w628 w632 w636 w640 w644 w648 w652 w656]
              tunnel: w614 -> [w627 w631 w635 w639 w643 w647 w651 w655]
              frame 1, Default {
                n148 = Bundle By Name(cluster=w630, "State"=w628, "Sensor1"=w627) -> (w629:T1)
              }
              frame 2 {
                n149 = Bundle By Name(cluster=w634, "State"=w632, "Sensor2"=w631) -> (w633:T1)
              }
              frame 3 {
                n150 = Bundle By Name(cluster=w638, "State"=w636, "Sensor3"=w635) -> (w637:T1)
              }
              frame 4 {
                n151 = Bundle By Name(cluster=w642, "State"=w640, "Sensor4"=w639) -> (w641:T1)
              }
              frame 5 {
                n152 = Bundle By Name(cluster=w646, "State"=w644, "Sensor5"=w643) -> (w645:T1)
              }
              frame 6 {
                n153 = Bundle By Name(cluster=w650, "State"=w648, "Sensor6"=w647) -> (w649:T1)
              }
              frame 7 {
                n154 = Bundle By Name(cluster=w654, "State"=w652, "Sensor7"=w651) -> (w653:T1)
              }
              frame 8 {
                n155 = Bundle By Name(cluster=w658, "State"=w656, "Sensor8"=w655) -> (w657:T1)
              }
            }
          }
        }
      }
      frame "ReadTenThousandths" {
        n156 = case shown="1, Default" w691 {
          tunnel: w690 -> [w697 _ _ _ _ _ _ _]
          tunnel: w689 -> [_ w698 _ _ _ _ _ _]
          tunnel: w688 -> [_ _ w699 _ _ _ _ _]
          tunnel: w687 -> [_ _ _ w700 _ _ _ _]
          tunnel: w686 -> [_ _ _ _ w701 _ _ _]
          tunnel: w685 -> [_ _ _ _ _ w702 _ _]
          tunnel: w684 -> [_ _ _ _ _ _ w703 _]
          tunnel: w683 -> [_ _ _ _ _ _ _ w704]
          tunnel: [w697 w698 w699 w700 w701 w702 w703 w704] -> w682
          frame 1, Default {
          }
          frame 2 {
          }
          frame 3 {
          }
          frame 4 {
          }
          frame 5 {
          }
          frame 6 {
          }
          frame 7 {
          }
          frame 8 {
          }
        }
        n157 = xnode ("FIFO Method Node")("Timeout"=0) -> ("Element"=w692:u8, "Timed Out?"=w693:bool)  [unwired: 1 in, 1 out]
        n158 = case shown="False" w693 {
          tunnel: w696 -> [w705 w723]
          tunnel: [w705 w722] -> w695
          tunnel: w692 -> [_ w721]
          tunnel: w691 -> [_ w718]
          tunnel: w682 -> [_ w713]
          tunnel: w681 -> [_ w707]
          frame True {
          }
          frame False {
            n159 = case shown="0, Default" w721 {
              tunnel: [0 0 1 2 3 4 5 6 7 8 9] -> w720
              tunnel: [FALSE TRUE TRUE TRUE TRUE TRUE TRUE TRUE TRUE TRUE TRUE] -> w717
              frame 0, Default {
                # "Invalid"
              }
              frame 48 {
                # "0"
              }
              frame 49 {
                # "1"
              }
              frame 50 {
                # "2"
              }
              frame 51 {
                # "3"
              }
              frame 52 {
                # "4"
              }
              frame 53 {
                # "5"
              }
              frame 54 {
                # "6"
              }
              frame 55 {
                # "7"
              }
              frame 56 {
                # "8"
              }
              frame 57 {
                # "9"
              }
            }
            n160 = Select(t=-1 ("x*y"), s=w707, f=1) -> (s? t:f=w708:i32)
            n161 = Multiply(x=w720, y=1) -> (x*y=w712:i32)
            n162 = Add(x=w713, y=w712) -> (x+y=w710:i32)
            n163 = Multiply(x=w710, y=w708) -> (x*y=w709:i32)
            n164 = Select(t=DisplacementStates."ReadDeliminator" ("State"), s=w717, f=DisplacementStates."ResponseInvalidError" ("State")) -> (s? t:f=w716:T2)
            n165 = case shown="1, Default" w718 {
              tunnel: w723 -> [w727 w731 w735 w739 w743 w747 w751 w755]
              tunnel: [w726 w730 w734 w738 w742 w746 w750 w754] -> w722
              tunnel: w716 -> [w725 w729 w733 w737 w741 w745 w749 w753]
              tunnel: w709 -> [w724 w728 w732 w736 w740 w744 w748 w752]
              frame 1, Default {
                n166 = Bundle By Name(cluster=w727, "State"=w725, "Sensor1"=w724) -> (w726:T1)
              }
              frame 2 {
                n167 = Bundle By Name(cluster=w731, "State"=w729, "Sensor2"=w728) -> (w730:T1)
              }
              frame 3 {
                n168 = Bundle By Name(cluster=w735, "State"=w733, "Sensor3"=w732) -> (w734:T1)
              }
              frame 4 {
                n169 = Bundle By Name(cluster=w739, "State"=w737, "Sensor4"=w736) -> (w738:T1)
              }
              frame 5 {
                n170 = Bundle By Name(cluster=w743, "State"=w741, "Sensor5"=w740) -> (w742:T1)
              }
              frame 6 {
                n171 = Bundle By Name(cluster=w747, "State"=w745, "Sensor6"=w744) -> (w746:T1)
              }
              frame 7 {
                n172 = Bundle By Name(cluster=w751, "State"=w749, "Sensor7"=w748) -> (w750:T1)
              }
              frame 8 {
                n173 = Bundle By Name(cluster=w755, "State"=w753, "Sensor8"=w752) -> (w754:T1)
              }
            }
          }
        }
      }
      frame "StartMoveData" {
        n174 = call "GetTelemetryUpdateDataConstant.vi"() -> ("TelemetryUpdateData"=w779:T9)  [unwired: 11 in]
        n175 = Bundle By Name(cluster=w779, "DataType"=TelemetryDataTypes."U64" ("TelemetryDataTypes"), "Mode"=TelemetryUpdateModes."+" ("TelemetryUpdateModes"), "Field"=TelemetryFields."DisplacementRxFrames", "Data"=u64 1) -> (w778:T9)
        n176 = xnode ("FIFO Method Node")("Element"=w778, "Timeout"=0) -> ()  [unwired: 1 in, 2 out]
        n177 = Bundle By Name(cluster=w788, "State"=DisplacementStates."MoveTimestamp", "Sensor"=u8 1) -> (w787:T1)
      }
      frame "MoveTimestamp" {
        n178 = call "GetTelemetryUpdateDataConstant.vi"() -> ("TelemetryUpdateData"=w791:T9)  [unwired: 11 in]
        n179 = Bundle By Name(cluster=w791, "DataType"=TelemetryDataTypes."U64" ("TelemetryDataTypes"), "Mode"=TelemetryUpdateModes."=" ("TelemetryUpdateModes"), "Field"=TelemetryFields."DisplacementTimestamp", "Data"=w789) -> (w790:T9)
        n180 = xnode ("FIFO Method Node")("Element"=w790, "Timeout"=0) -> ()  [unwired: 1 in, 2 out]
        n181 = Bundle By Name(cluster=w799, "State"=DisplacementStates."MoveData", "Sensor"=u8 1) -> (w798:T1)
      }
      frame "MoveData" {
        n182 = case shown="1, Default" w807 {
          tunnel: w821 -> [w824 _ _ _ _ _ _ _]
          tunnel: w820 -> [_ w826 _ _ _ _ _ _]
          tunnel: w819 -> [_ _ w828 _ _ _ _ _]
          tunnel: w818 -> [_ _ _ w830 _ _ _ _]
          tunnel: w817 -> [_ _ _ _ w832 _ _ _]
          tunnel: w816 -> [_ _ _ _ _ w834 _ _]
          tunnel: w815 -> [_ _ _ _ _ _ w836 _]
          tunnel: w814 -> [_ _ _ _ _ _ _ w838]
          tunnel: [w824 w826 w828 w830 w832 w834 w836 w838] -> w802
          tunnel: [TelemetryFields."Displacement1" ("TelemetryFields") TelemetryFields."Displacement2" ("TelemetryFields") TelemetryFields."Displacement3" ("TelemetryFields") TelemetryFields."Displacement4" ("TelemetryFields") TelemetryFields."Displacement5" ("TelemetryFields") TelemetryFields."Displacement6" ("TelemetryFields") TelemetryFields."Displacement7" ("TelemetryFields") TelemetryFields."Displacement8" ("TelemetryFields")] -> w801
          frame 1, Default {
          }
          frame 2 {
          }
          frame 3 {
          }
          frame 4 {
          }
          frame 5 {
          }
          frame 6 {
          }
          frame 7 {
          }
          frame 8 {
          }
        }
        n183 = call "GetTelemetryUpdateDataConstant.vi"() -> ("TelemetryUpdateData"=w803:T9)  [unwired: 11 in]
        n184 = Bundle By Name(cluster=w803, "DataType"=TelemetryDataTypes."I32" ("TelemetryDataTypes"), "Mode"=TelemetryUpdateModes."=" ("TelemetryUpdateModes"), "Field"=w801, "Data"=w802) -> (w800:T9)
        n185 = Equal?(x=w807, y=u8 8) -> (x = y?=w809:bool)
        n186 = Increment(x=w807) -> (x+1=w806:u8)
        n187 = xnode ("FIFO Method Node")("Element"=w800, "Timeout"=0) -> ()  [unwired: 1 in, 2 out]
        n188 = Select(t=DisplacementStates."WaitForTrigger" ("State"), s=w809, f=DisplacementStates."MoveData" ("State")) -> (s? t:f=w813:T2)
        n189 = Bundle By Name(cluster=w823, "State"=w813, "Sensor"=w806) -> (w822:T1)
      }
      frame "ReadErrorResponse" {
        n190 = Bundle By Name(cluster=w842, "State"=DisplacementStates."WaitForTrigger") -> (w841:T1)
      }
      frame "ResponseUnknownError" {
        w843 = T10 1 items=["None"=0, "ResponseUnknownError"=1, "ResponseInvalidError"=2, "ResponseTimeoutError"=4] ("DisplacementErrorCodes")
        n191 = call "GetTelemetryUpdateDataConstant.vi"() -> ("TelemetryUpdateData"=w845:T9)  [unwired: 11 in]
        n192 = Bundle By Name(cluster=w845, "DataType"=TelemetryDataTypes."U8" ("TelemetryDataTypes"), "Mode"=TelemetryUpdateModes."=" ("TelemetryUpdateModes"), "Field"=TelemetryFields."DisplacementErrorCode", "Data"=w843) -> (w844:T9)
        n193 = xnode ("FIFO Method Node")("Element"=w844, "Timeout"=0) -> ()  [unwired: 1 in, 2 out]
        n194 = Bundle By Name(cluster=w852, "State"=DisplacementStates."WaitForTrigger") -> (w851:T1)
      }
      frame "ResponseInvalidError" {
        w854 = T10 2 items=["None"=0, "ResponseUnknownError"=1, "ResponseInvalidError"=2, "ResponseTimeoutError"=4] ("DisplacementErrorCodes")
        n195 = call "GetTelemetryUpdateDataConstant.vi"() -> ("TelemetryUpdateData"=w855:T9)  [unwired: 11 in]
        n196 = Bundle By Name(cluster=w855, "DataType"=TelemetryDataTypes."U8" ("TelemetryDataTypes"), "Mode"=TelemetryUpdateModes."=" ("TelemetryUpdateModes"), "Field"=TelemetryFields."DisplacementErrorCode", "Data"=w854) -> (w853:T9)
        n197 = xnode ("FIFO Method Node")("Element"=w853, "Timeout"=0) -> ()  [unwired: 1 in, 2 out]
        n198 = Bundle By Name(cluster=w862, "State"=DisplacementStates."WaitForTrigger") -> (w861:T1)
      }
    }
  }
  n199 = node-c288(w2) -> ()
